vi "New Fruit.vi"(6 "Color Box":u32(colorbox), 8 "error in (no error)":errorcluster) -> (0 "error out":errorcluster, 3 "Fruit out":refnum<class "Fruit.lvclass">)   [LabVIEW 2018, in "Fruit.lvclass"]
uses:
  Fruit.lvclass
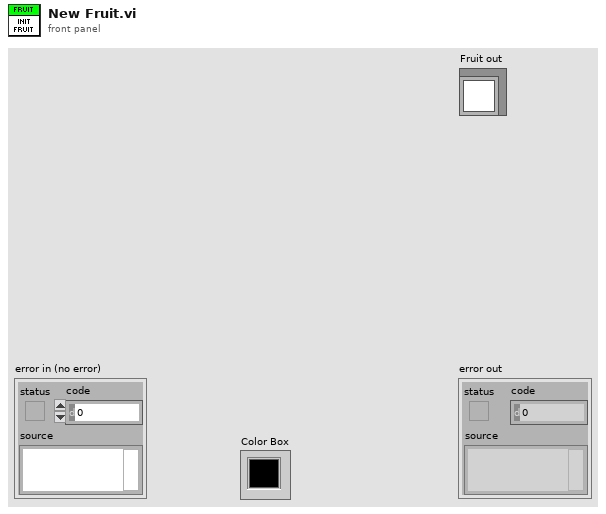
[diagram p1: front panel]
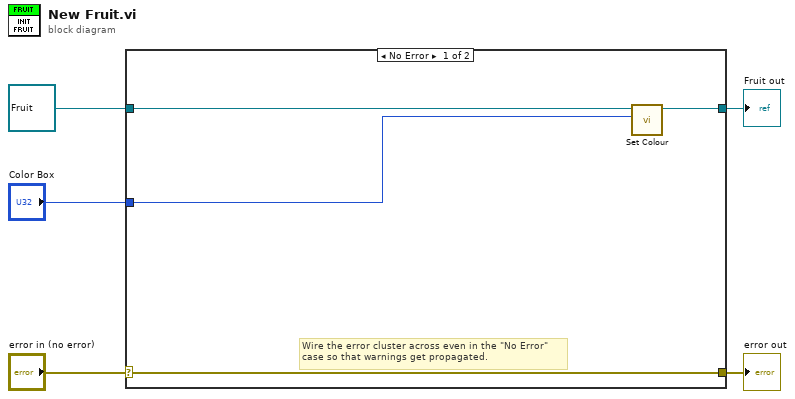
[diagram p0: block diagram]
diagram:
  n1 = case shown="No Error" "error in (no error)" {
    selector: "error in (no error)" -> [w9 w11]
    tunnel: [w9 w11] -> w4
    tunnel: [w7 w10] -> w2
    tunnel: refnum<class "Fruit.lvclass"> refnum ("Fruit in") -> [w8 w10]
    tunnel: "Color Box" -> [w6 _]
    frame No Error {
      # "Wire the error cluster across even in the \"No Error\"\ncase so that warnings get propagated."
      n2 = call-dynamic "Set Colour.vi"("Componant Colour"=w6, "Game Componants in"=w8) -> ("Game Componants out"=w7:refnum<class "Fruit.lvclass">)  [unwired: 9 in]
    }
    frame Error {
    }
  }
  "error out" <- w4
  "Fruit out" <- w2
